vi "send action report.vi"(8 "error in":errorcluster, 9 "command error":errorcluster, 10 "commands":T1, 11 "message queue in":T2) -> (0 "error out":errorcluster, 3 "message queue out":T2)   [LabVIEW 2013, in "DCAF Execution Service.lvlib"]
uses:
  DCAF Execution Service.lvlib
  <vilib>/NI/AMC/Message Queue.ctl
  <vilib>/NI/AMC/Message.ctl
  <vilib>/NI/Tools/Keyed Array/KeyedArray.ctl
  command commands to rtexe process.ctl
  common reponses to network process.ctl
  <vilib>/NI/AMC/Create Single Message.vi
  <vilib>/NI/AMC/Update Message Routing Info.vi
  <vilib>/NI/AMC/Send Message.vi
  <vilib>/NI/AMC/AMC.lvlib
  <vilib>/NI/Tools/Keyed Array/Tools_KeyedArray.lvlib
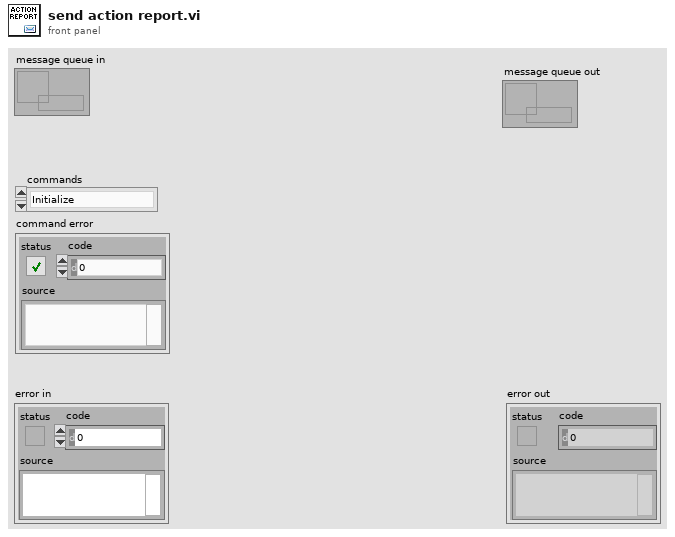
[diagram p1: front panel]
types:
  T1 = typedef "DCAF Execution Service.lvlib/command commands to rtexe process.ctl" = enum16{"Initialize", "Add Search Paths", "Load from File", "Unload File", "Open All Engines", "Open Single Engine", "Initialize All Engines", "Initialize Single Engine", "Start All", "Start Single", "Pause All", "Pause Single", "Stop All", "Stop Single", "Close All", "Close Single", "Set Safe State All", "Set Safe State Single", "Get Status", "Exit", "Error", "Load Bitfile", "Unload Bitfile", "Clear Faults Single", "Clear Faults All"}
  T2 = typedef "AMC.lvlib/Message Queue.ctl" = refnum<queue>
  T3 = typedef "DCAF Execution Service.lvlib/common reponses to network process.ctl" = enum16{"System Error", "Load Report", "Action Response", "Engine Status"}
  T4 = cluster{"command string":string, "command error":errorcluster}
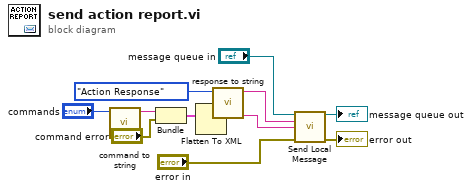
[diagram p0: block diagram]
diagram:
  n1 = call "command to string.vi"("commands"="commands") -> ("command string"=w7:string)  [unwired: 10 in]
  n2 = Bundle("command string"=w7, "command error"="command error") -> (w3:T4)  [unwired: 1 in]
  n3 = Flatten To XML(anything=w3) -> (xml string=w2:string)
  n4 = call "response to string.vi"("responses"=common_reponses_to_network_process."Action Response") -> ("command string"=w5:string)  [unwired: 10 in]
  n5 = call <vilib>:"Send Local Message.vi"("message queue in"="message queue in", "message name"=w5, "message value"=w2, "error in"="error in") -> ("message queue out"=→"message queue out":T2, "error out"=→"error out":errorcluster)  [unwired: 9 in, 1 out]
